vi "SetChannels.vi"(8 "error in (no error)":errorcluster, 10 "Channels":T1, 11 "IviFgen in":refnum<class "IviFgen.lvclass">) -> (0 "error out":errorcluster, 3 "IviFgen out":refnum<class "IviFgen.lvclass">)   [LabVIEW 2014, in "FgenPlugins.lvlib" / "IviFgen.lvclass"]
uses:
  IviFgen.lvclass
  TypeDefs/Channels.ctl
  TypeDefs/Channel.ctl
  FgenPluginBaseClass/FgenPluginsBase.lvclass/FgenPluginsBase.ctl
  FgenPluginBaseClass/Accessors/Read Channels.vi
  FgenPluginBaseClass/FgenPluginsBase.lvclass
  FgenPlugins.lvlib
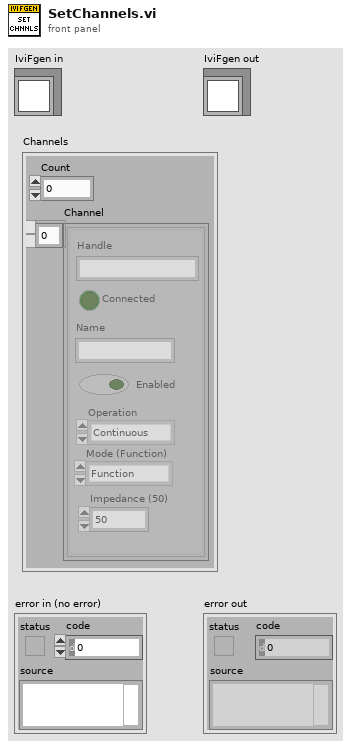
[diagram p1: front panel]
types:
  T1 = typedef "FgenPlugins.lvlib/Channels.ctl" = cluster{"Count":u16, "Channel":T2[]}
  T2 = typedef "FgenPlugins.lvlib/Channel.ctl" = cluster{"Name":string, "Enabled":bool, "Operation":enum16{"Continuous", "Burst"}, "Impedance (50)":dbl, "Handle":string, "Connected":bool, "Mode (Function)":enum16{"Function", "Arbitrary", "Sequence"}}
  T3 = typedef "Channel.ctl" = cluster{"Name":string, "Enabled":bool, "Operation":enum16{"Continuous", "Burst"}, "Impedance (50)":dbl, "Handle":string, "Connected":bool, "Mode (Function)":enum16{"Function", "Arbitrary", "Sequence"}}
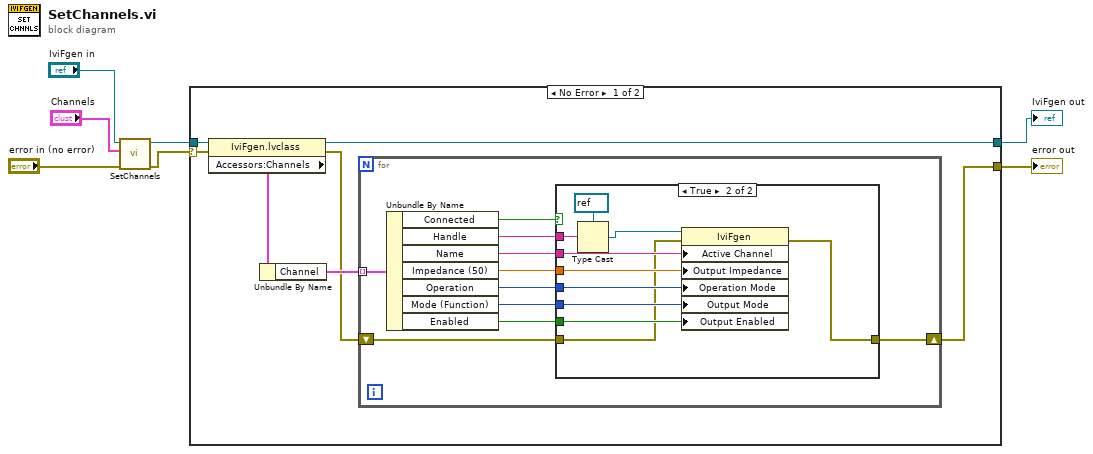
[diagram p0: block diagram]
diagram:
  n1 = call-parent "SetChannels.vi"("error in (no error)"="error in (no error)", "Channels"="Channels", "FgenPluginsBase in"="IviFgen in") -> ("error out"=w2:errorcluster, "FgenPluginsBase out"=w7:refnum<class "IviFgen.lvclass">)  [unwired: 7 in]
  n2 = case shown="No Error" w2 {
    selector: w2 -> [w12 w36]
    tunnel: w7 -> [w14 w37]
    tunnel: [w13 w37] -> w3
    tunnel: [w9 w36] -> w1
    frame No Error {
      n3 = property class="IviFgen.lvclass"(reference=w14, error in=w12) -> (reference out=w13:refnum<class "IviFgen.lvclass">, error out=w8:errorcluster, "Accessors:Channels"=w11:cluster{"Count":u16, "Channel":T3[]})
      n4 = Unbundle By Name(w11) -> ("Channel"=w10:T3[])
      n5 = for {
        tunnel: w10 -> [w24] mode=indexing
        shift-right: [w15] -> w9
        shift-left: w8 -> [w19]
        n6 = Unbundle By Name(w24) -> ("Connected"=w23:bool, "Handle"=w22:string, "Name"=w21:string, "Impedance (50)"=w20:dbl, "Operation"=w18:enum16{"Continuous", "Burst"}, "Mode (Function)"=w17:enum16{"Function", "Arbitrary", "Sequence"}, "Enabled"=w16:bool)
        n7 = case shown="True" w23 {
          tunnel: w22 -> [_ w35]
          tunnel: w21 -> [_ w32]
          tunnel: w20 -> [_ w31]
          tunnel: w18 -> [_ w30]
          tunnel: w17 -> [_ w29]
          tunnel: w16 -> [_ w28]
          tunnel: w19 -> [w25 w27]
          tunnel: [w25 w26] -> w15
          frame False {
          }
          frame True {
            n8 = Type Cast(type=refnum<k15> refnum ("reference"), x=w35) -> (*(type *) &x=w33:refnum<k15>)
            n9 = property class="IviFgen"(reference=w33, error in=w27, "Active Channel"=w32, "Output Impedance"=w31, "Operation Mode"=w30, "Output Mode"=w29, "Output Enabled"=w28) -> (error out=w26:errorcluster)  [unwired: 1 out]
          }
        }
      }
    }
    frame Error {
    }
  }
  "error out" <- w1
  "IviFgen out" <- w3
